vi "GOOP_ClassTemplateLookup.vi"(10 "ClassType":string, 11 "ClassTemplateFolderIn":path) -> (3 "ClassTemplateFolderOut":path)   [LabVIEW 2012]
uses:
  <vilib>/Utility/config.llb/Read Key (Path).vi
  <vilib>/Utility/config.llb/NI_LVConfig.lvlib
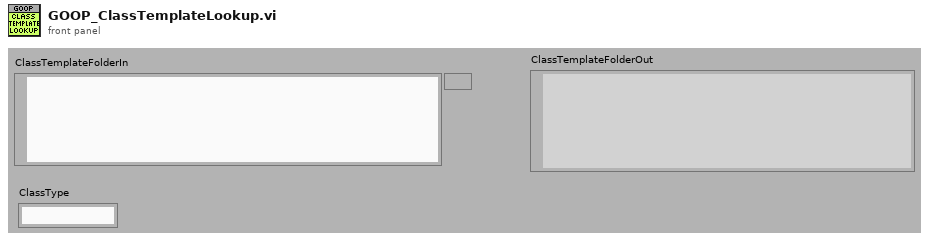
[diagram p1: front panel]
types:
  T1 = typedef "NI_LVConfig.lvlib/Config Data RefNum.ctl" = refnum<k1>
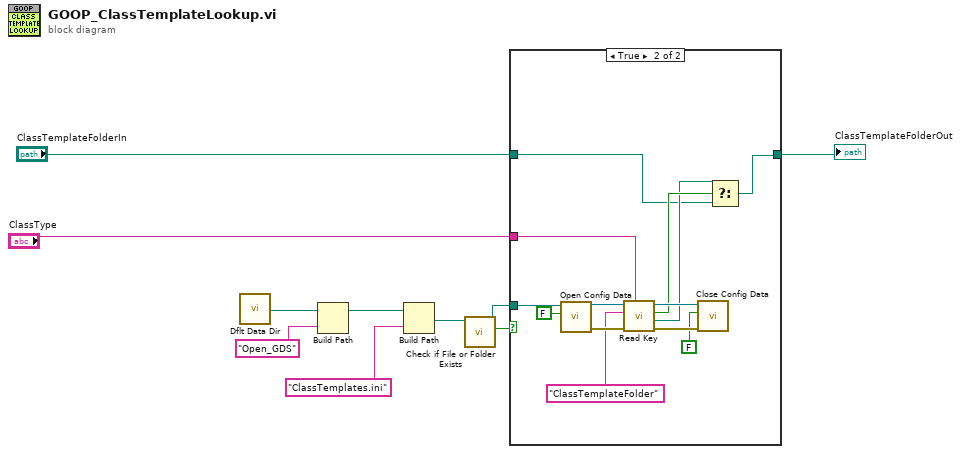
[diagram p0: block diagram]
diagram:
  n1 = call <vilib>:"Dflt Data Dir.vi"() -> ("App:Default Data Directory"=w10:path)
  n2 = Build Path(base path=w10, name or relative path="Open_GDS") -> (appended path=w8:path)
  n3 = Build Path(base path=w8, name or relative path="ClassTemplates.ini") -> (appended path=w6:path)
  n4 = call <vilib>:"Check if File or Folder Exists.vi"("path"=w6) -> ("file or folder exists?"=w5:bool, "dup path"=w4:path)  [unwired: 8 in, 1 out]
  n5 = case shown="True" w5 {
    tunnel: w4 -> [_ w21]
    tunnel: "ClassType" -> [_ w20]
    tunnel: "ClassTemplateFolderIn" -> [w11 w14]
    tunnel: [w11 w13] -> w1
    frame False {
    }
    frame True {
      n6 = call <vilib>:"Open Config Data.vi"("create file if necessary (T)"=FALSE, "configuration file path"=w21) -> ("error out"=w23:errorcluster, "refnum"=w24:T1)  [unwired: 7 in, 1 out]
      n7 = call-poly <vilib>:"Read Key.vi"("section"=w20, "error in (no error)"=w23, "key"="ClassTemplateFolder", "refnum"=w24) -> ("error out"=w17:errorcluster, "value"=w15:path, "found?"=w16:bool, "refnum out"=w18:T1)  [unwired: 4 in]
      n8 = call <vilib>:"Close Config Data.vi"("error in (no error)"=w17, "write file if changed (T)"=FALSE ("create file if necessary (T)"), "refnum"=w18) -> ()  [unwired: 7 in, 2 out]
      n9 = Select(t=w15, s=w16, f=w14) -> (s? t:f=w13:path)
    }
  }
  "ClassTemplateFolderOut" <- w1
